vi "capture.vi"(4 "PWM frames (0, auto)":u32, 5 "Capture Range (0, auto)":u32, 6 "isPWM (no)":bool, 7 "VISA resource name":refnum<visa-resource-name>="ASRL13::INSTR") -> (2 "Error":bool, 3 "dup VISA resource name":refnum<visa-resource-name>="ASRL13::INSTR")   [LabVIEW 2020, in "Library Instrument & Equipement.lvlib" / "Library LED Analyser.lvlib"]
uses:
  Library LED Analyser.lvlib
panel:
  in  "Error":bool
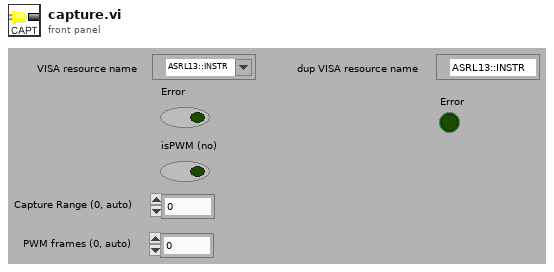
[diagram p1: front panel]
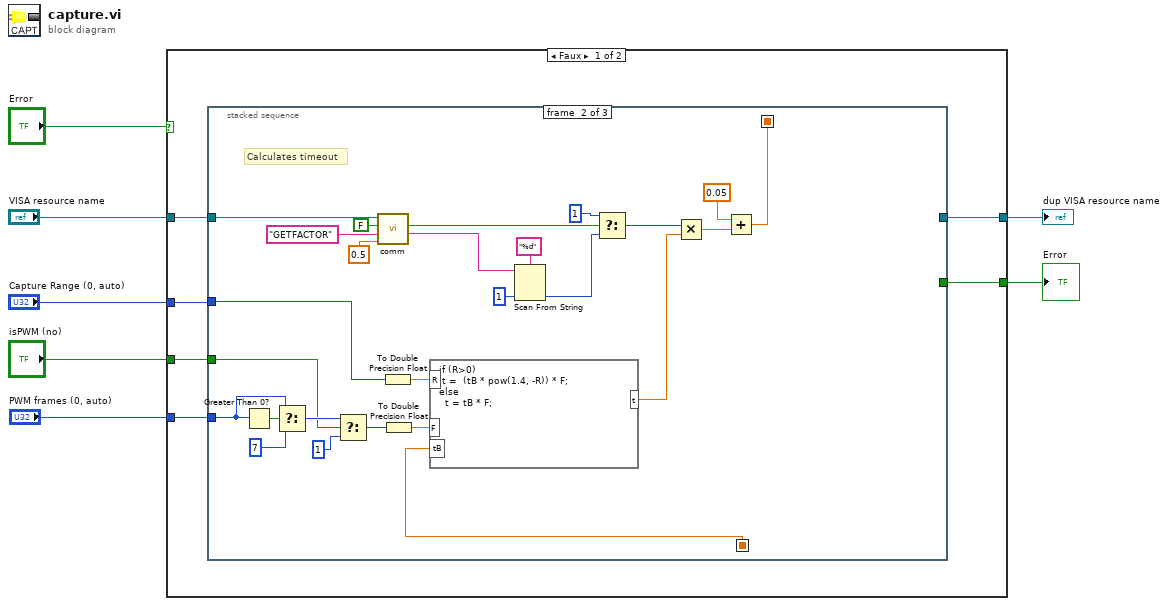
[diagram p0: block diagram]
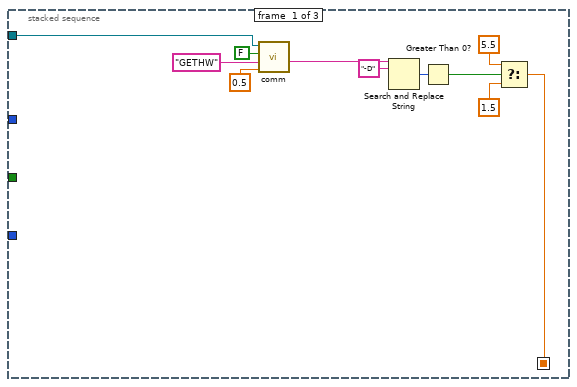
[diagram p2: hidden frame]
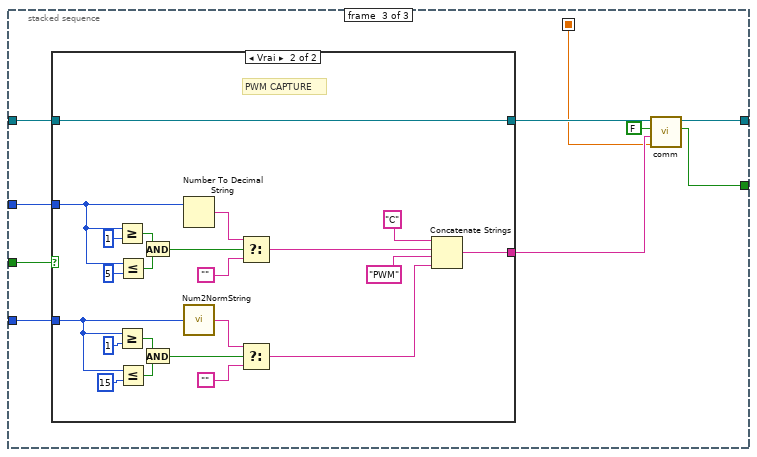
[diagram p3: hidden frame]
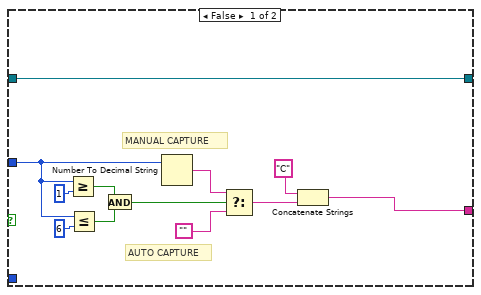
[diagram p4: hidden frame]
diagram:
  n1 = case shown="Faux" "Error" {
    selector: "Error" -> [_ w96]
    tunnel: "Capture Range (0, auto)" -> [w13 _]
    tunnel: "VISA resource name" -> [w12 w95]
    tunnel: "PWM frames (0, auto)" -> [w11 _]
    tunnel: "isPWM (no)" -> [w10 _]
    tunnel: [w9 w95] -> w3
    tunnel: [w8 w96] -> w1
    frame False {
      n2 = stacked-sequence {
        seq-local: [w15 _ _] -> [_ w32 _]
        seq-local: [_ w31 _] -> [_ _ w52]
        tunnel: w13 -> [_ w25 w60]
        tunnel: w12 -> [w14 w50 w59]
        tunnel: w11 -> [_ w38 w58]
        tunnel: w10 -> [_ w35 w57]
        tunnel: [_ _ w54] -> w9
        tunnel: [_ _ w51] -> w8
        frame #0 {
          n3 = call "comm.vi"("Timeout (s)"=0.5, "Command"="GETHW", "Error"=FALSE, "VISA resource name"=w14) -> ("Response"=w20:string)  [unwired: 2 in, 3 out]
          n4 = Search and Replace String(input string=w20, search string="-D") -> (number of replacements=w18:i32)  [unwired: 6 in, 3 out]
          n5 = Greater Than 0?(x=w18) -> (x > 0?=w16:bool)
          n6 = Select(t=5.5, s=w16, f=1.5) -> (s? t:f=w15:dbl)
        }
        frame #1 {
          # "Calculates timeout"
          n7 = Greater Than 0?(x=w38) -> (x > 0?=w39:bool)
          n8 = Select(t=w38, s=w39, f=u32 7) -> (s? t:f=w36:u32)
          n9 = Select(t=w36, s=w35, f=u32 1) -> (s? t:f=w27:u32)
          n10 = call "comm.vi"("Timeout (s)"=0.5, "Command"="GETFACTOR", "Error"=FALSE, "VISA resource name"=w50) -> ("Response"=w44:string, "Error"=w46:bool)  [unwired: 2 in, 2 out]
          n11 = To Double Precision Float(number=w25) -> (double precision float=w28:dbl)
          n12 = To Double Precision Float(number=w27) -> (double precision float=w26:dbl)
          n13 = formula code="if (R>0)\n t =  (tB * pow(1.4, -R)) * F;\nelse\n  t = tB * F;"("R"=w28, "F"=w26, "tB"=w32) -> ("t"=w33:dbl)
          n14 = Scan From String(format string="%d", input string=w44, default 1=1 ("default value 1")) -> (output 1=w42:i32)  [unwired: 2 in, 3 out]
          n15 = Select(t=1, s=w46, f=w42) -> (s? t:f=w34:i32)
          n16 = Multiply(x=w34, y=w33) -> (x*y=w30:dbl)
          n17 = Add(x=0.05, y=w30) -> (x+y=w31:dbl)
        }
        frame #2 {
          n18 = case shown="Vrai" w57 {
            tunnel: [w72 w89] -> w55
            tunnel: w60 -> [w64 w76]
            tunnel: w59 -> [w65 w87]
            tunnel: [w65 w87] -> w56
            tunnel: w58 -> [_ w85]
            frame False {
              # "AUTO CAPTURE"
              # "MANUAL CAPTURE"
              n19 = Greater Or Equal?(x=w64, y=1) -> (x >= y?=w67:bool)
              n20 = Less Or Equal?(x=w64, y=6) -> (x <= y?=w66:bool)
              n21 = And(x=w67, y=w66) -> (x .and. y?=w68:bool)
              n22 = Number To Decimal String(number=w64) -> (decimal integer string=w63:string)  [unwired: 1 in]
              n23 = Select(t=w63, s=w68, f="") -> (s? t:f=w61:string)
              n24 = Concatenate Strings("C" ("Command"), w61) -> (w72:string)
            }
            frame True {
              # "PWM CAPTURE"
              n25 = Greater Or Equal?(x=w76, y=1) -> (x >= y?=w79:bool)
              n26 = Greater Or Equal?(x=w85, y=1) -> (x >= y?=w92:bool)
              n27 = Less Or Equal?(x=w76, y=5) -> (x <= y?=w78:bool)
              n28 = Less Or Equal?(x=w85, y=15) -> (x <= y?=w91:bool)
              n29 = And(x=w79, y=w78) -> (x .and. y?=w77:bool)
              n30 = And(x=w92, y=w91) -> (x .and. y?=w86:bool)
              n31 = Number To Decimal String(number=w76) -> (decimal integer string=w75:string)  [unwired: 1 in]
              n32 = call "Num2NormString.vi"("Number"=w85) -> ("Normalized String Number"=w84:string)
              n33 = Select(t=w75, s=w77, f="") -> (s? t:f=w73:string)
              n34 = Select(t=w84, s=w86, f="") -> (s? t:f=w82:string)
              n35 = Concatenate Strings("C", w73, "PWM", w82) -> (w89:string)
            }
          }
          n36 = call "comm.vi"("Timeout (s)"=w52, "Command"=w55, "Error"=FALSE, "VISA resource name"=w56) -> ("Error"=w51:bool, "dup VISA resource name"=w54:refnum<visa-resource-name>)  [unwired: 2 in, 2 out]
        }
      }
    }
    frame True {
    }
  }
  "dup VISA resource name" <- w3
  "Error" <- w1
